vi "ts_M1M3ThermalFPGA.vi"() -> ()   [LabVIEW 2023]
uses:
  Utility/TelemetryStatistics.ctl
  Common_FPGA_HealthAndStatus/DataTypes/HealthAndStatusFIFOCopySettings.ctl
  Common_FPGA_HealthAndStatus/DataTypes/HealthAndStatusSettings.ctl
  Common_FPGA_Modbus/DataTypes/ModbusPortSettings.ctl
  <vilib>/rvi/Emulation/niFpgaGetClockAttributes.vi
  <vilib>/rvi/Emulation/niFpgaSctlEmulationGetInTimedLoop.vi
  <vilib>/rvi/Emulation/niFpgaEmulationReportErrorSimple.vi
  <vilib>/rvi/eio/common/nirviEmuTemplateMethod_errors.vi
  <vilib>/rvi/Emulation/niFpgaCriticalErrorInLSC.vi
  <vilib>/eio/EIOMethodNode/EIOMethodNode.xnode
  Common_FPGA_HealthAndStatus/FPGAHealthAndStatus.lvlib
  Common_FPGA_Modbus/FPGAModbus.lvlib
panel:
  out "Flow Meter Timeout":bool
  out "Flow Meter Read":u64
  out "Flow Meter Transmitted":u64
  out "Glycool Timeout":bool
  out "Glycool Read":u64
  out "Glycool Transmitted":u64
  out "Chassis Temperature":fxp<+/-,32,16>
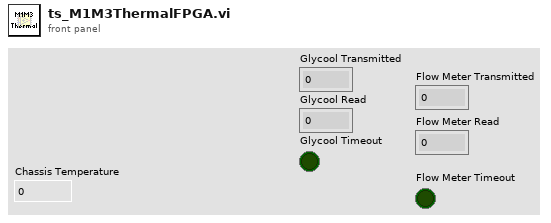
[diagram p1: front panel]
types:
  T1 = typedef "FPGAModbus.lvlib/ModbusPortSettings.ctl" = cluster{"TxPort":refnum<k21>, "TxDataFIFO":refnum<k21>, "TxInternalDataFIFO":refnum<k21>, "TxHealthAndStatusFIFO":refnum<k21>, "RxPort":refnum<k21>, "RxDataFIFO":refnum<k21>, "RxHealthAndStatusFIFO":refnum<k21>, "WaitForRxFrameRegister":refnum<k21>, "BaseHealthAndStatusAddress":u32, "IRQAddress":u8, "TriggerIRQRegister":refnum<k21>, "SoftwareControlledTrigger":refnum<k21>, "TimestampRegister":refnum<k21>, "TxTimestampFIFO":refnum<k21>}
  T2 = typedef "FPGAHealthAndStatus.lvlib/HealthAndStatusSettings.ctl" = cluster{"InternalHealthAndStatusFIFO":refnum<k21>, "HealthAndStatusQueryFIFO":refnum<k21>, "HealthAndStatusResponseFIFO":refnum<k21>, "HealthAndStatusMemory":refnum<k21>, "MemorySize":i32}
  T3 = typedef "FPGAHealthAndStatus.lvlib/HealthAndStatusFIFOCopySettings.ctl" = cluster{"InternalHealthAndStatusFIFO":refnum<k21>, "SourceHealthAndStatusFIFO":refnum<k21>}
  T4 = typedef "TelemetryStatistics.ctl" = cluster{"Transmited":u64, "Received":u64, "Timeout":bool}
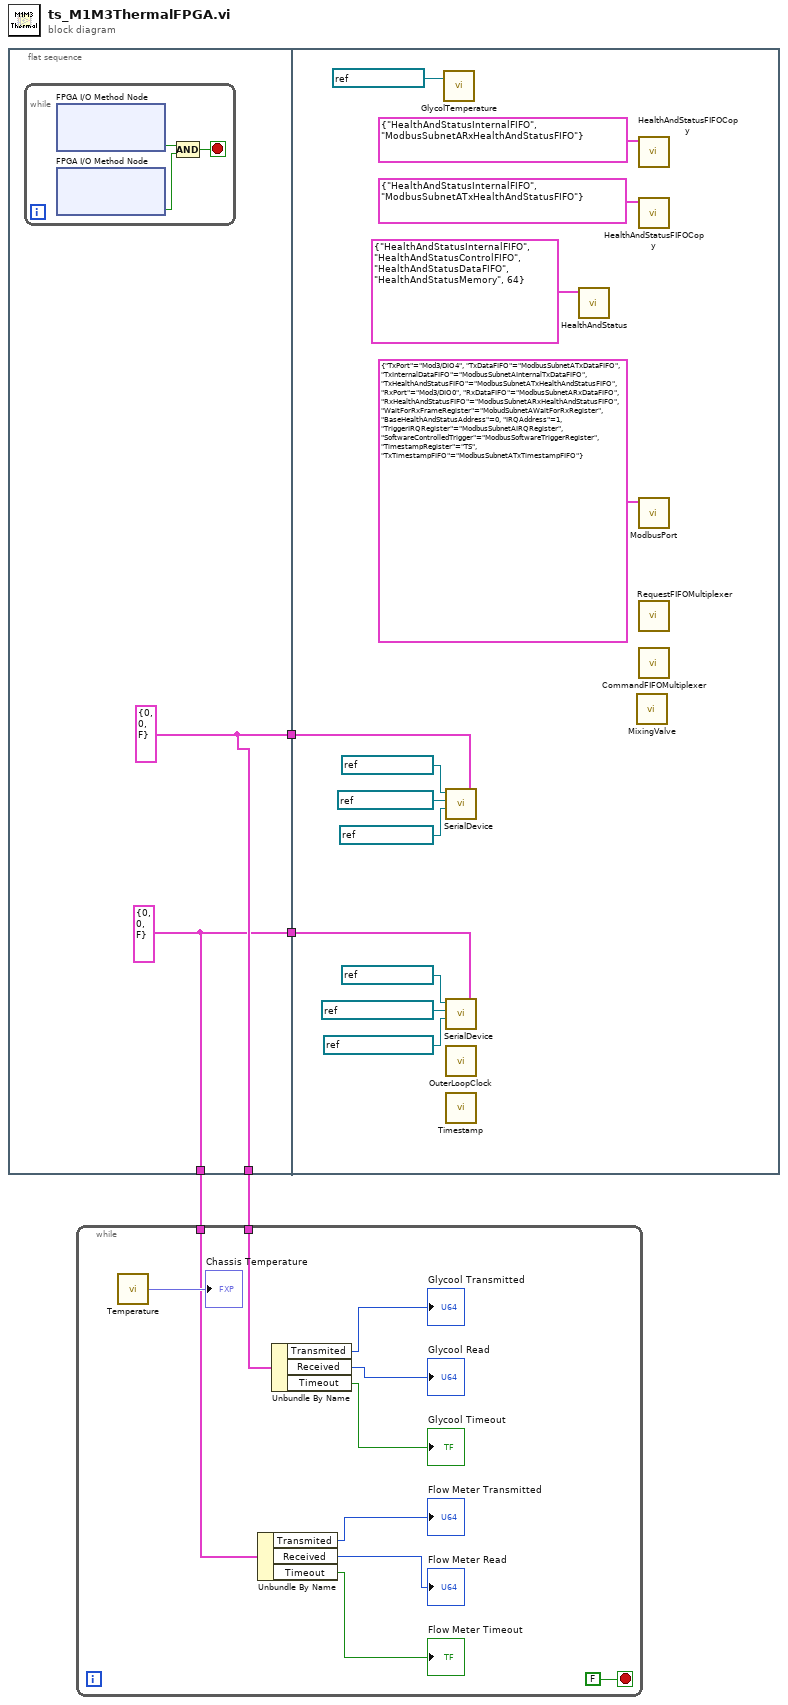
[diagram p0: block diagram]
diagram:
  n1 = flat-sequence {
    tunnel: [w5] -> w4
    tunnel: [w6] -> w3
    tunnel: [w6] -> w2
    tunnel: [w5] -> w1
    tunnel: w4 -> [w11]
    tunnel: w3 -> [w10]
    frame #0 {
      w5 = T4 {"Transmited"=0, "Received"=0, "Timeout"=FALSE} ("TelemetryStatistics")
      w6 = T4 {"Transmited"=0, "Received"=0, "Timeout"=FALSE} ("TelemetryStatistics")
      n2 = while {
        stop <- w7 stop-if-true
        n3 = xnode "FPGA I/O Method Node"() -> ("Ready"=w9:bool)  [unwired: 1 in, 1 out]
        n4 = xnode "FPGA I/O Method Node"() -> ("Ready"=w8:bool)  [unwired: 1 in, 1 out]
        n5 = Compound Arithmetic op=AND(w9, w8) -> (w7:bool)
      }
    }
    frame #1 {
      n6 = call "GlycolTemperature.vi"("cRIO I/O Device"=refnum<k21> "Mod7\\Port1") -> ()  [unwired: 2 in]
      n7 = call "SerialDevice.vi"("TelemetryStatistics"=w10, "Out"=refnum<k21> "GlycoolRead", "In"=refnum<k21> "GlycoolWrite", "Port"=refnum<k21> "Mod6\\Port1") -> ()  [unwired: 3 in, 1 out]
      n8 = call "SerialDevice.vi"("TelemetryStatistics"=w11, "Out"=refnum<k21> "FlowMeterRead", "In"=refnum<k21> "FlowMeterWrite", "Port"=refnum<k21> "Mod6\\Port2") -> ()  [unwired: 3 in, 1 out]
      n9 = call "OuterLoopClock.vi"() -> ()  [unwired: 12 in]
      n10 = call "Timestamp.vi"() -> ()  [unwired: 12 in]
      n11 = call "HealthAndStatus.vi"("HealthAndStatusSettings"=T2 {"InternalHealthAndStatusFIFO"="HealthAndStatusInternalFIFO", "HealthAndStatusQueryFIFO"="HealthAndStatusControlFIFO", "HealthAndStatusResponseFIFO"="HealthAndStatusDataFIFO", "HealthAndStatusMemory"="HealthAndStatusMemory", "MemorySize"=64}) -> ()  [unwired: 11 in]
      n12 = call "MixingValve.vi"() -> ()  [unwired: 12 in]
      n13 = call "HealthAndStatusFIFOCopy.vi"("HealthAndStatusSettingsFIFOCopySettings"=T3 {"InternalHealthAndStatusFIFO"="HealthAndStatusInternalFIFO", "SourceHealthAndStatusFIFO"="ModbusSubnetARxHealthAndStatusFIFO"}) -> ()  [unwired: 11 in]
      n14 = call "HealthAndStatusFIFOCopy.vi"("HealthAndStatusSettingsFIFOCopySettings"=T3 {"InternalHealthAndStatusFIFO"="HealthAndStatusInternalFIFO", "SourceHealthAndStatusFIFO"="ModbusSubnetATxHealthAndStatusFIFO"}) -> ()  [unwired: 11 in]
      n15 = call "ModbusPort.vi"("ModbusPortSettings"=T1 {"TxPort"="Mod3/DIO4", "TxDataFIFO"="ModbusSubnetATxDataFIFO", "TxInternalDataFIFO"="ModbusSubnetAInternalTxDataFIFO", "TxHealthAndStatusFIFO"="ModbusSubnetATxHealthAndStatusFIFO", "RxPort"="Mod3/DIO0", "RxDataFIFO"="ModbusSubnetARxDataFIFO", "RxHealthAndStatusFIFO"="ModbusSubnetARxHealthAndStatusFIFO", "WaitForRxFrameRegister"="MobudSubnetAWaitForRxRegister", "BaseHealthAndStatusAddress"=0, "IRQAddress"=1, "TriggerIRQRegister"="ModbusSubnetAIRQRegister", "SoftwareControlledTrigger"="ModbusSoftwareTriggerRegister", "TimestampRegister"="TS", "TxTimestampFIFO"="ModbusSubnetATxTimestampFIFO"}) -> ()  [unwired: 10 in]
      n16 = call "RequestFIFOMultiplexer.vi"() -> ()  [unwired: 12 in]
      n17 = call "CommandFIFOMultiplexer.vi"() -> ()  [unwired: 12 in]
    }
  }
  n18 = while {
    tunnel: w2 -> [w30]
    tunnel: w1 -> [w26]
    stop <- FALSE stop-if-true
    n19 = call "Temperature.vi"() -> ("Mean temperature"=→"Chassis Temperature":fxp<+/-,32,16>)  [unwired: 1 in]
    n20 = Unbundle By Name(w26) -> ("Transmited"=→"Flow Meter Transmitted":u64, "Received"=→"Flow Meter Read":u64, "Timeout"=→"Flow Meter Timeout":bool)
    n21 = Unbundle By Name(w30) -> ("Transmited"=→"Glycool Transmitted":u64, "Received"=→"Glycool Read":u64, "Timeout"=→"Glycool Timeout":bool)
  }
